vi "rqcBob Get Detector State (2 SPD).vi"(0 "rqcBob HW Control in":T1, 1 "clock in":bool) -> (4 "rqcBob HW Control out":T1, 8 "SPD state":u16, 15 "write to fifo":bool)   [LabVIEW 2018]
uses:
  Custom Controls/rqcBob HW Control.ctl
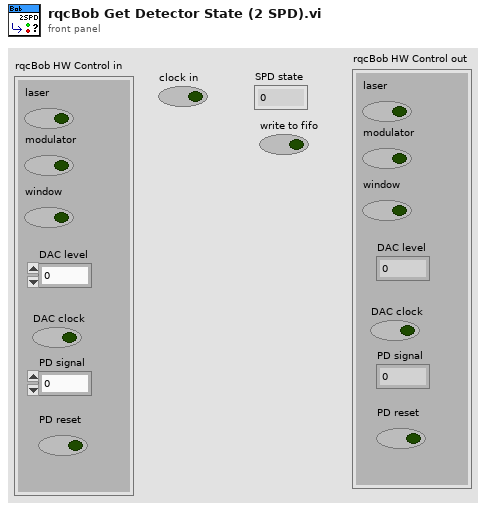
[diagram p1: front panel]
types:
  T1 = typedef "rqcBob HW Control.ctl" = cluster{"laser":bool, "modulator":bool, "window":bool, "DAC level":u8, "DAC clock":bool, "PD signal":u8, "PD reset":bool}
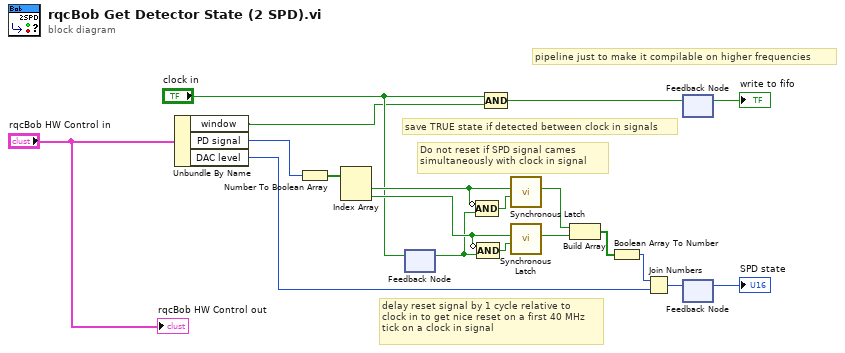
[diagram p0: block diagram]
diagram:
  # "delay reset signal by 1 cycle relative to \nclock in to get nice reset on a first 40 MHz\ntick on a clock in signal"
  # "Do not reset if SPD signal cames \nsimultaneously with clock in signal"
  # "save TRUE state if detected between clock in signals"
  # "pipeline just to make it compilable on higher frequencies"
  n1 = Unbundle By Name("rqcBob HW Control in") -> ("window"=w1:bool, "PD signal"=w4:u8, "DAC level"=w3:u8)
  n2 = Number To Boolean Array(number=w4) -> (Boolean array=w6:bool[])
  n3 = Index Array(array=w6) -> (element #1=w11:bool, element #2=w9:bool)  [unwired: 2 in]
  n4 = feedback #1() -> (w7:bool)  [unwired: 1 in]
  n5 = feedback-in #1("clock in") -> ()
  n6 = Compound Arithmetic op=AND(invert w11, w7) -> (w10:bool)
  n7 = Compound Arithmetic op=AND(invert w9, w7) -> (w8:bool)
  n8 = Compound Arithmetic op=AND("clock in", w1) -> (w19:bool)
  n9 = call <vilib>:"Synchronous Latch.vi"("clear"=w10, "set"=w11) -> ("out"=w18:bool)  [unwired: 9 in]
  n10 = call <vilib>:"Synchronous Latch.vi"("clear"=w8, "set"=w9) -> ("out"=w15:bool)  [unwired: 9 in]
  n11 = Build Array(w18, w15) -> (w17:bool[])
  n12 = Boolean Array To Number(Boolean array=w17) -> (number=w16:u8)
  n13 = Join Numbers(hi=w16, lo=w3) -> ((hi.lo)=w13:u16)
  n14 = feedback #2() -> (→"write to fifo":bool)  [unwired: 1 in]
  n15 = feedback-in #2(w19) -> ()
  n16 = feedback #3() -> (→"SPD state":u16)  [unwired: 1 in]
  n17 = feedback-in #3(w13) -> ()
  "rqcBob HW Control out" <- "rqcBob HW Control in"
